vi "Tektronix_scope_Daniel.vi"() -> ()   [LabVIEW 2020]
doc: "This example illustrates how to use autosetup and continuously acquires waveforms from a single channel using the following steps:\n\n1. Specify a valid VISA session. \n2. Specify a channel. \n3. Specify a time-out value for reading waveform.\n4. Run the VI. The graph displays the waveform you acquire."
uses:
  <instrlib>/Tektronix DPO MSO 2000 4000 Series/Public/Data/Read (Multiple Waveforms).vi
  <instrlib>/Tektronix DPO MSO 2000 4000 Series/Tektronix DPO MSO 2000 4000 Series.lvlib
panel:
  out "Waveform Graph":waveform(dbl)[](graph)
  in  "Channels":u16[](array[ring]) items=["Channel 1", "Channel 2", "Channel 3", "Channel 4", "Math", "Reference 1", "Reference 2", "Reference 3", "Reference 4", "D0", "D1", "D2", "D3", "D4", "D5", "D6", "D7", "D8", "D9", "D10", "D11", "D12", "D13", "D14", "D15", "Amplitude", "Frequency", "Phase", "Normal", "Average", "Maximum Peak Hold", "Minimum Peak Hold"]
  in  "stop":bool
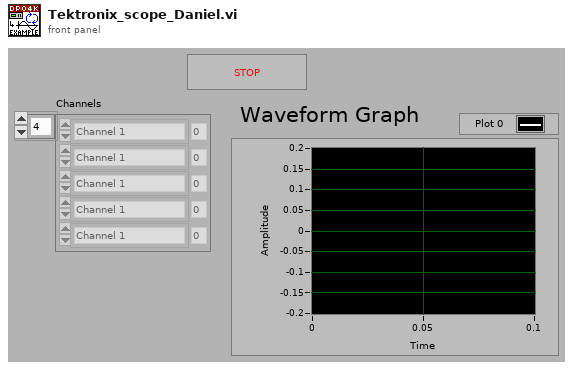
[diagram p1: front panel]
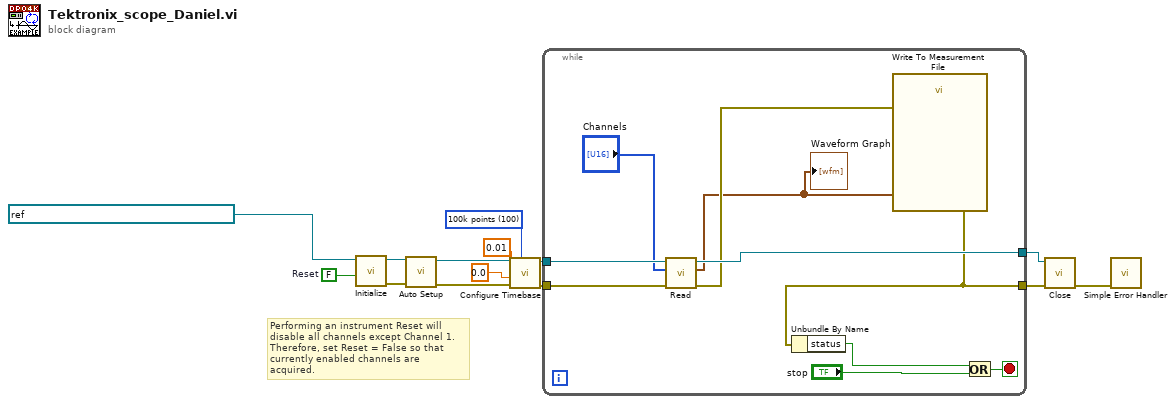
[diagram p0: block diagram]
diagram:
  w4 = u32 100 items=["1000 points"=1, "10k points"=10, "100k points"=100, "1M points"=1000, "5M points"=5000, "10M points"=10000] ("Record Length (10: 10k points)")
  w11 = FALSE  # Reset
  # "Performing an instrument Reset will disable all channels except Channel 1. Therefore, set Reset = False so that currently enabled channels are acquired."
  n1 = call <instrlib>:"Initialize.vi"("Reset (True)"=w11, "VISA resource name"=refnum<visa-resource-name> "USB0::0x0699::0x0421::C010309::INSTR" ("VISA Resource Name")) -> ("error out"=w12:errorcluster, "VISA resource name out"=w13:refnum<visa-resource-name>)  [unwired: 8 in]
  n2 = call <instrlib>:"Auto Setup.vi"("error in (no error)"=w12, "VISA resource name"=w13) -> ("error out"=w8:errorcluster, "VISA resource name out"=w9:refnum<visa-resource-name>)  [unwired: 8 in]
  n3 = call <instrlib>:"Configure Timebase.vi"("Record Length (10: 10k points)"=w4, "error in (no error)"=w8, "Position (10 %)"=0.0, "Timebase (0.0005 s)"=0.01, "VISA resource name"=w9) -> ("error out"=w7:errorcluster, "VISA resource name out"=w10:refnum<visa-resource-name>)  [unwired: 5 in]
  n4 = while {
    tunnel: w10 -> [w23]
    tunnel: w7 -> [w22]
    tunnel: [w18] -> w2
    tunnel: [w20] -> w1
    stop <- w24 stop-if-true
    n5 = call-poly <instrlib>:"Read.vi"("error in (no error)"=w22, "Channels"="Channels", "VISA resource name"=w23) -> ("error out"=w17:errorcluster, "Waveform Data"=w15:waveform(dbl)[], "VISA resource name out"=w20:refnum<visa-resource-name>)  [unwired: 6 in]
    "Waveform Graph" <- w15
    n6 = call "Write To Measurement File"("Signals"=w15, "error in (no error)"=w17) -> ("error out"=w18:errorcluster)  [unwired: 15 in, 2 out]
    n7 = Unbundle By Name(w18) -> ("status"=w19:bool)
    n8 = Or(x=w19, y="stop") -> (x .or. y?=w24:bool)
  }
  n9 = call <instrlib>:"Close.vi"("error in (no error)"=w2, "VISA resource name"=w1) -> ("error out"=w14:errorcluster)  [unwired: 9 in]
  n10 = call <vilib>:"Simple Error Handler.vi"("error in (no error)"=w14) -> ()  [unwired: 4 in, 5 out]
